vi "CAN R&W.vi"(0 "设备类型":u32(ring)=4 items=["PCI5121"=1, "PCI9810"=2, "USBCAN1"=3, "USBCAN2"=4, "PCI9820"=5, "CAN232"=6, "PCI5110"=7, "CANLite(mini)"=8, "ISA9620"=9, "ISA5420"=10, "PC104CAN"=11, "CANETE"=12, "DNP9810"=13], 1 "设备索引":u32(ring) items=["0", "1", "2", "3", "4", "5", "6", "7", "8", "9", "10", "11", "12", "13", "14", "15", ""], 2 "CAN路数":u32(ring) items=["0", "1"], 3 "DataLen":u8, 4 "写地址/数据":enum16{"写地址", "写数据"}(ring), 5 "Data Input":string, 6 "枚举":enum16{"请选择板类型", "主板", "从板", "高压板"}(ring), 7 "错误输入（无错误）":errorcluster, 8 "TYPE":string, 9 "queue out":refnum<queue>) -> (20 "发送的数据":i32[](array[numeric]), 27 "错误输出":errorcluster)   [LabVIEW 2013]
uses:
  Settings/ControlCAN.dll
panel:
  out "VCI_CAN_OBJ_T 2":T1 {"ID" format="%x"}
  out "VCI_CAN_OBJ_T":T1 {"ID" format="%x"}
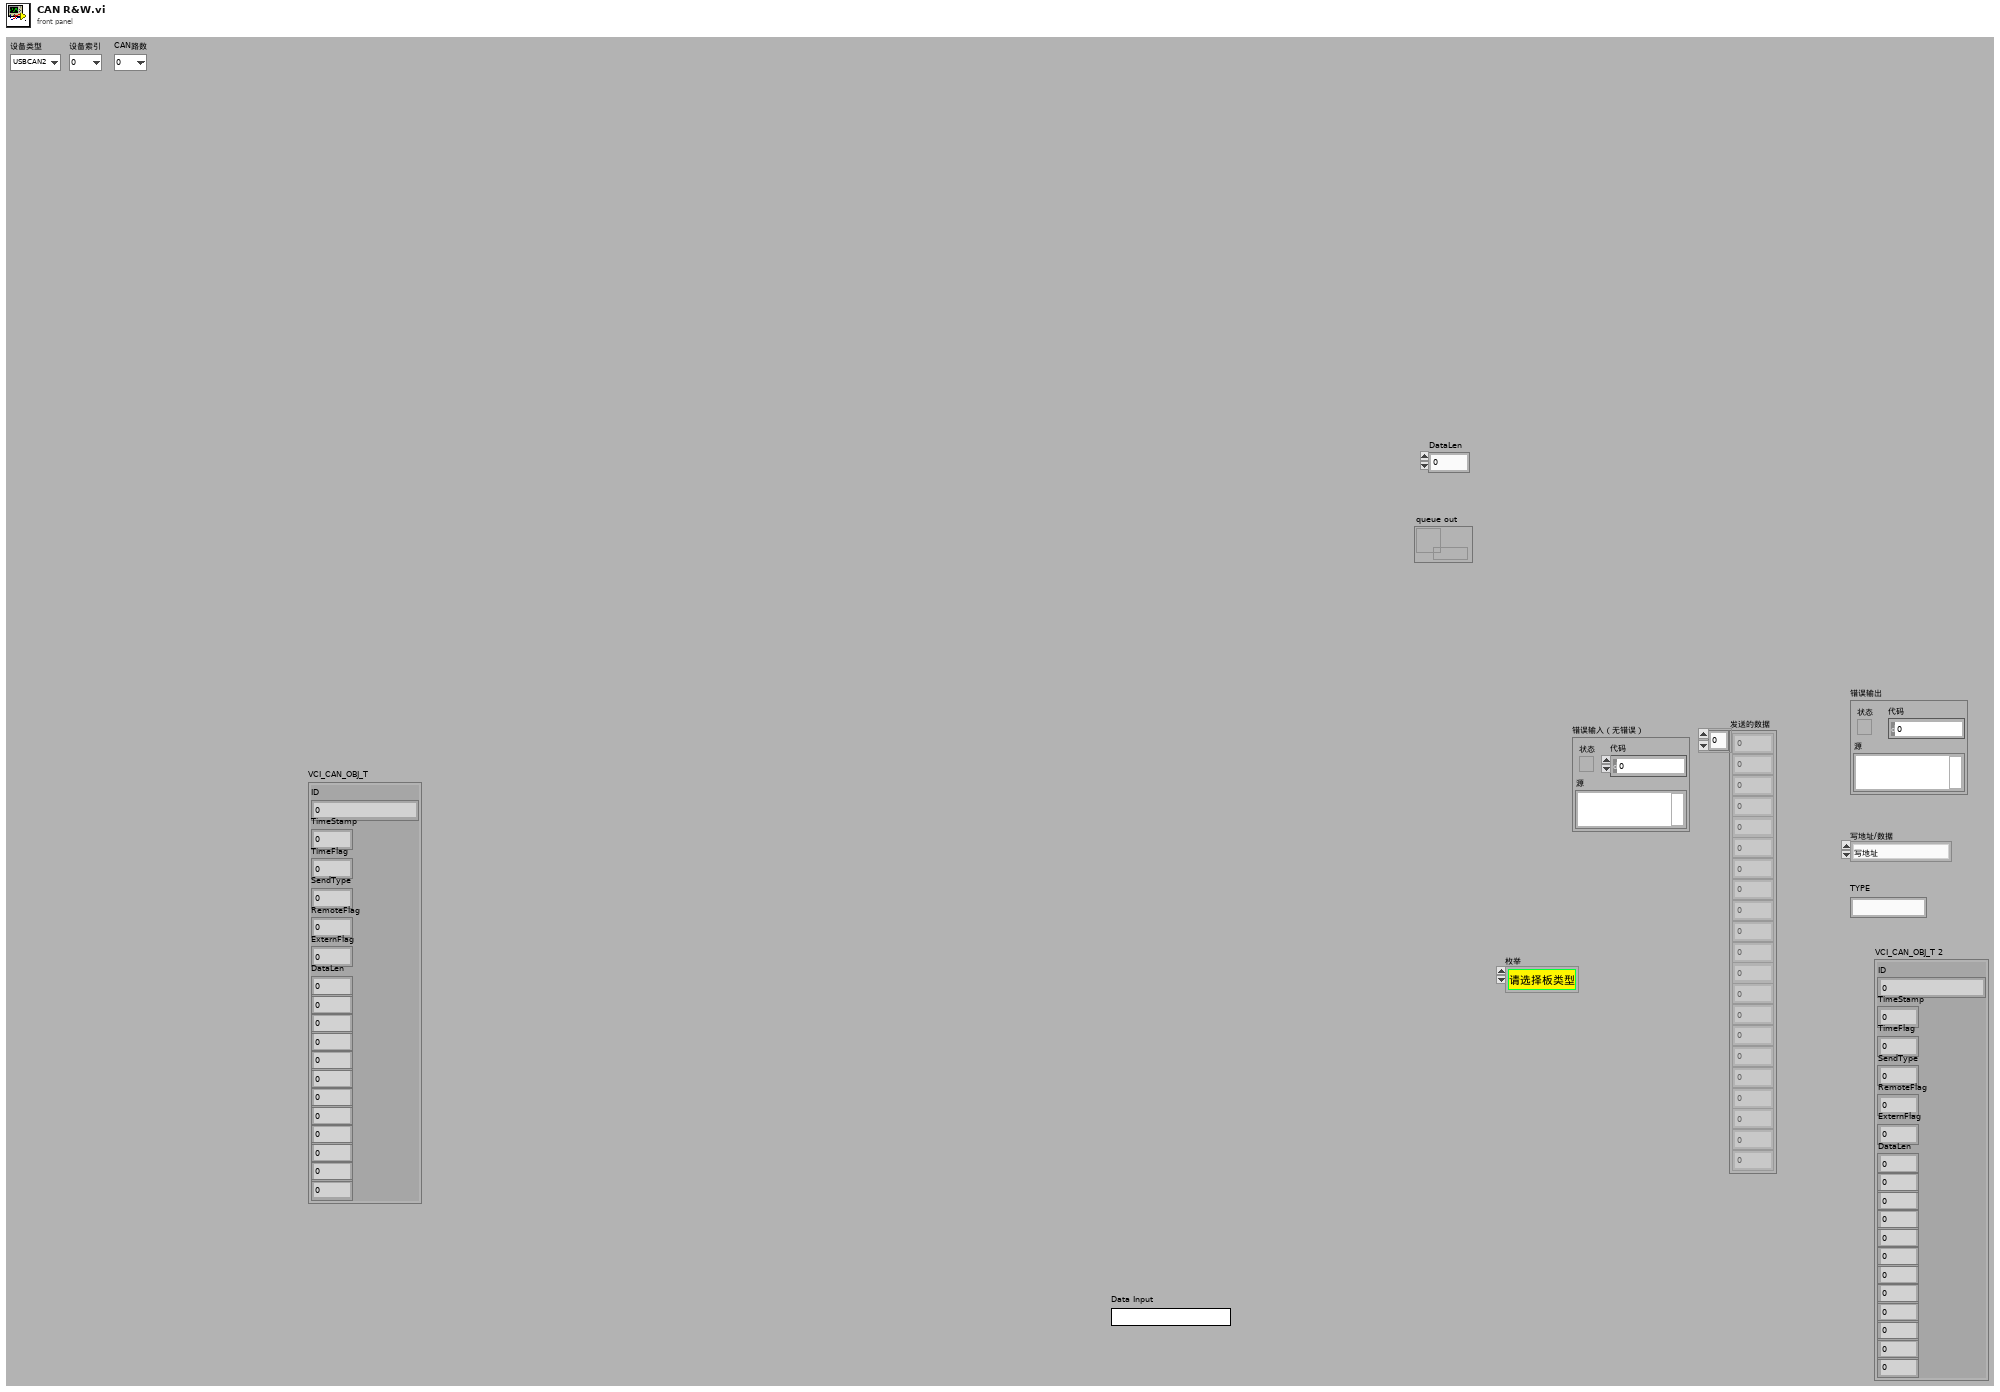
[diagram p1: front panel]
types:
  T1 = cluster{"ID":u32, "TimeStamp":u32, "TimeFlag":u8, "SendType":u8, "RemoteFlag":u8, "ExternFlag":u8, "DataLen":u8, u8, u8, u8, u8, u8, u8, u8, u8, u8, u8, u8}
  T2 = cluster{"[0]":u32, "[1]":u32, "[2]":u32, "[3]":u32, "[4]":u32, "[5]":u32}
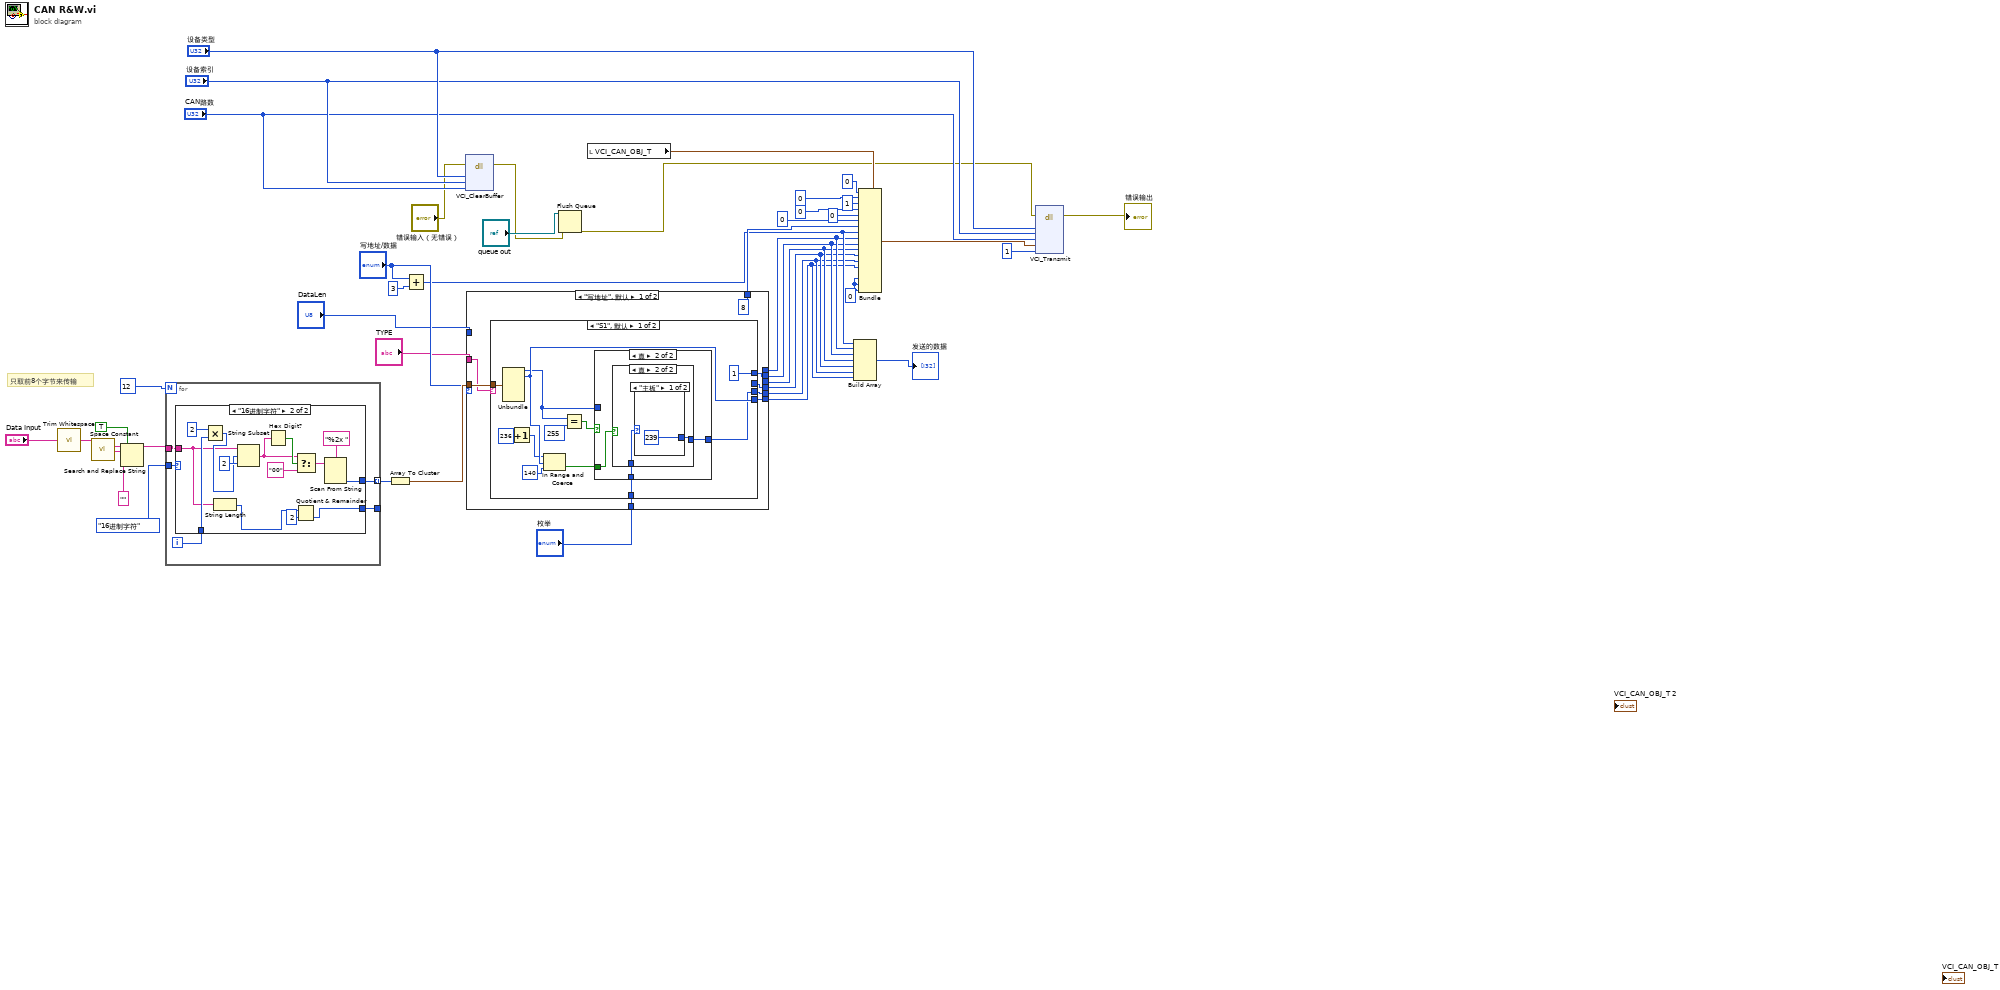
[diagram p0: block diagram]
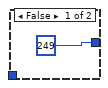
[diagram p3: hidden frame]
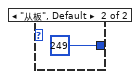
[diagram p4: hidden frame]
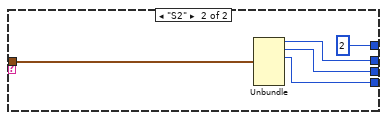
[diagram p5: hidden frame]
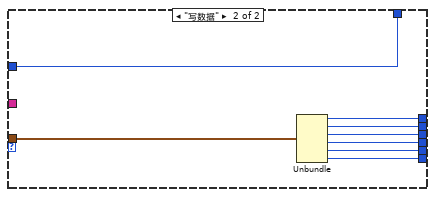
[diagram p6: hidden frame]
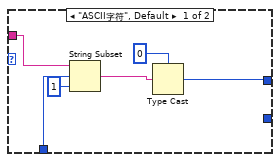
[diagram p7: hidden frame]
diagram:
  w27 = u8 0 ("元素")
  # "只取前8个字节来传输"
  n1 = call <vilib>:"Trim Whitespace.vi"("string"="Data Input") -> ("trimmed string"=w36:string)  [unwired: 1 in]
  n2 = call <vilib>:"Space Constant.vi"() -> ("String"=w35:string)
  n3 = Search and Replace String(replace all?=TRUE ("替换全部？(F)"), input string=w36, search string=w35, replace string="" ("替换字符串(\"\")")) -> (result string=w32:string)  [unwired: 1 in, 6 out]
  n4 = for {
    N: 12 -> [_]
    tunnel: w32 -> [w45]
    tunnel: [w47] -> w40 mode=indexing
    tunnel: [w44] -> _
    tunnel: enum16{"ASCII字符", "16进制字符"}."16进制字符" ("传入类型") -> [w43]
    i -> [w46]
    n5 = case shown="\"16进制字符\"" w43 {
      tunnel: [w48 w64] -> w47
      tunnel: w46 -> [w51 w59]
      tunnel: w45 -> [w53 w57]
      tunnel: [_ w54] -> w44
      frame "ASCII字符", Default {
        n6 = String Subset(string=w53, offset (0)=w51, length (rest)=1 ("长度（剩余）")) -> (substring=w49:string)
        n7 = Type Cast(type=u8 0, x=w49) -> (*(type *) &x=w48:u8)
      }
      frame "16进制字符" {
        n8 = Multiply(x=2, y=w59) -> (x*y=w58:i32)
        n9 = String Length(string=w57) -> (length=w56:i32)
        n10 = String Subset(string=w57, offset (0)=w58, length (rest)=2 ("length (rest)")) -> (substring=w61:string)
        n11 = Hex Digit?(1:w61) -> (0:w62:bool)
        n12 = Select(t=w61, s=w62, f="00" ("t")) -> (s? t:f=w63:string)
        n13 = Quotient & Remainder(x=w56, y=2) -> (floor(x/y)=w54:i32)  [unwired: 1 out]
        n14 = Scan From String(format string="%2x ", input string=w63) -> (output 1=w64:u32)  [unwired: 2 in, 4 out]
      }
    }
  }
  n15 = Array To Cluster(array=w40) -> (cluster=w39:T2)
  n16 = Add(x="写地址/数据", y=u8 3 ("ExternFlag")) -> (x+y=w15:u16)
  n17 = dll-call lib="PTH1habs CUsersT450DesktopBMU_BootloaderG128应用程序下载器v1.0.0SettingsControlCAN.dll" fn="VCI_ClearBuffer" label="VCI_Clearbuffer"(error in="错误输入（无错误）", "DeviceType"="设备类型", "DeviceInd"="设备索引", "CANInd"="CAN路数") -> (error out=w3:errorcluster)  [unwired: 3 in, 4 out]
  n18 = case shown="\"写地址\", 默认" "写地址/数据" {
    tunnel: w39 -> [w75 w109]
    tunnel: [_ w108] -> w14
    tunnel: [w70 w107] -> w12
    tunnel: [_ w106] -> w11
    tunnel: [w71 w105] -> w10
    tunnel: [w73 w104] -> w9
    tunnel: [w72 w103] -> w8
    tunnel: "TYPE" -> [w74 _]
    tunnel: [u8 8 ("DataLen") w102] -> w18
    tunnel: "DataLen" -> [_ w102]
    tunnel: "枚举" -> [w68 _]
    frame "写地址", Default {
      n19 = case shown="\"S1\", 默认" w74 {
        tunnel: w75 -> [w87 w101]
        tunnel: [w80 w99] -> w73
        tunnel: [w83 w98] -> w72
        tunnel: [_ w100] -> w71
        tunnel: [u8 1 ("ExternFlag") u8 2 ("ExternFlag")] -> w70
        tunnel: w68 -> [w76 _]
        frame "S1", Default {
          n20 = Unbundle(w87) -> ("[0]"=w79:u32, "[1]"=w83:u32)  [unwired: 4 out]
          n21 = Increment(x=236 ("上限")) -> (x+1=w77:i32)
          n22 = In Range and Coerce(upper limit=w77, x=w83, lower limit=140 ("上限")) -> (In Range?=w81:bool)  [unwired: 1 out]
          n23 = Equal?(x=w79, y=255) -> (x = y?=w85:bool)
          n24 = case shown="真" w85 {
            tunnel: w81 -> [_ w91]
            tunnel: [w88 w90] -> w80
            tunnel: w79 -> [w88 _]
            tunnel: w76 -> [_ w89]
            frame False {
            }
            frame True {
              n25 = case shown="真" w91 {
                tunnel: [249 ("上限") w93] -> w90
                tunnel: w89 -> [_ w94]
                frame False {
                }
                frame True {
                  n26 = case shown="\"主板\"" w94 {
                    tunnel: [239 ("上限") 249 ("上限")] -> w93
                    frame "主板" {
                    }
                    frame "从板", Default {
                    }
                  }
                }
              }
            }
          }
        }
        frame "S2" {
          n27 = Unbundle(w101) -> ("[0]"=w100:u32, "[1]"=w99:u32, "[2]"=w98:u32)  [unwired: 3 out]
        }
      }
    }
    frame "写数据" {
      n28 = Unbundle(w109) -> ("[0]"=w108:u32, "[1]"=w107:u32, "[2]"=w106:u32, "[3]"=w105:u32, "[4]"=w104:u32, "[5]"=w103:u32)
    }
  }
  n29 = Flush Queue(queue="queue out", error in (no error)=w3) -> (error out=w1:errorcluster)  [unwired: 2 out]
  n30 = local read "VCI_CAN_OBJ_T"() -> (w23:T1)
  n31 = Build Array(w15, w14, w12, w11, w10, w9, w8) -> (→"发送的数据":u32[])
  n32 = Bundle(cluster=w23, "ID"=u32 0, "TimeStamp"=u8 0 ("RemoteFlag"), "TimeFlag"=u8 1, "SendType"=u8 0 ("DataLen"), "RemoteFlag"=u8 0, "ExternFlag"=u8 0, "DataLen"=w18, w15, w14, w12, w11, w10, w9, w8, w27, w27, w27) -> (w24:T1)  [unwired: 1 in]
  n33 = dll-call lib="PTH1habs CUsersT450DesktopBMU_BootloaderG128应用程序下载器v1.0.0SettingsControlCAN.dll" fn="VCI_Transmit"(error in=w1, "DeviceType"="设备类型", "DeviceInd"="设备索引", "CANInd"="CAN路数", "pSend"=w24, "Len"=u32 1) -> (error out=→"错误输出":errorcluster)  [unwired: 4 in, 5 out]
